vi "Fetch Power Measurement CCDF Percentiles.vi"(8 "error in (no error)":errorcluster, 10 "Instance (1)":i32=1, 11 "VISA resource name":refnum<visa-resource-name>) -> (0 "error out":errorcluster, 1 "Percentiles":dbl[](array[numeric]) format="%^.3e", 2 "Reliability":i32, 3 "VISA resource name out":refnum<visa-resource-name>)   [LabVIEW 2015, in "Rohde&Schwarz CMXP GPRF.lvlib"]
doc: "This VI returns percentiles of the complementary cumulative distribution VI (CCDF). This result is only available in \"Statistic\" evaluation mode (rscmwgprf Configure Power Measurement Result Mode.vi).\n\nAttribute:\nRSCMXPGPRF_ATTR_FETCH_POWER_MEASUREMENT_CCDF_PERCENTILES\n\nRemote-control command:\nFETCh:GPRF:MEAS<i>:POWer:CCDF:PROBability?"
uses:
  <instrlib>/Rohde&Schwarz CMXP GPRF/Rohde&Schwarz CMXP GPRF.lvlib
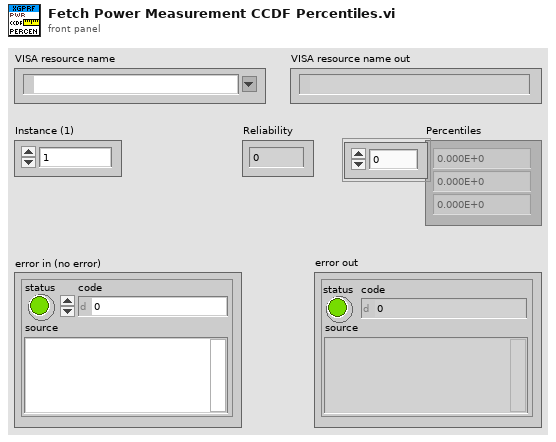
[diagram p1: front panel]
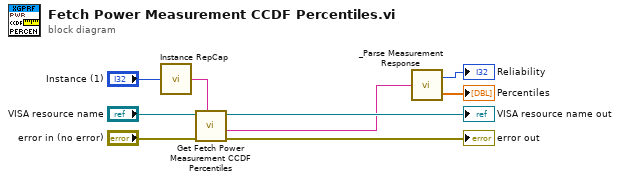
[diagram p0: block diagram]
diagram:
  n1 = call <instrlib>:"Instance RepCap.vi"("instance  in"="Instance (1)") -> ("instance out"=w4:string)
  n2 = call "Get Fetch Power Measurement CCDF Percentiles"("Repeated Capabilities"=w4, "error in (no error)"="error in (no error)", "instrument handle"="VISA resource name") -> ("error out"=→"error out":errorcluster, "Fetch Power Measurement CCDF Percentiles"=w1:string, "instrument handle out"=→"VISA resource name out":refnum<visa-resource-name>)  [unwired: 6 in]
  n3 = call <instrlib>:"_Parse Measurement Response.vi"("String In"=w1) -> ("Reliability"=→"Reliability":i32, "Data"=→"Percentiles":dbl[])
